vi "Load user settings.vi"(8 "error in (no error)":errorcluster, 11 "Test Framework in":refnum<class "Test Framework.lvclass">) -> (0 "error out":errorcluster, 2 "Canceled":bool, 3 "Test Framework out":refnum<class "Test Framework.lvclass">)   [LabVIEW 2020, in "Test Framework.lvclass"]
uses:
  Test Framework.lvclass
panel:
  in  "Cancel Button":bool
  in  "OK Button":bool caption="Restarts the framework"
  in  "User system setting file":path
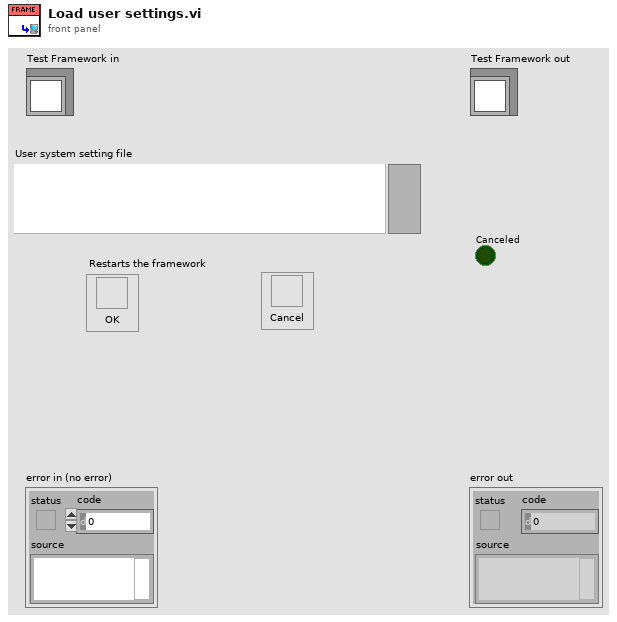
[diagram p1: front panel]
types:
  T1 = cluster{"Restart?":bool, "User system setting file":path}
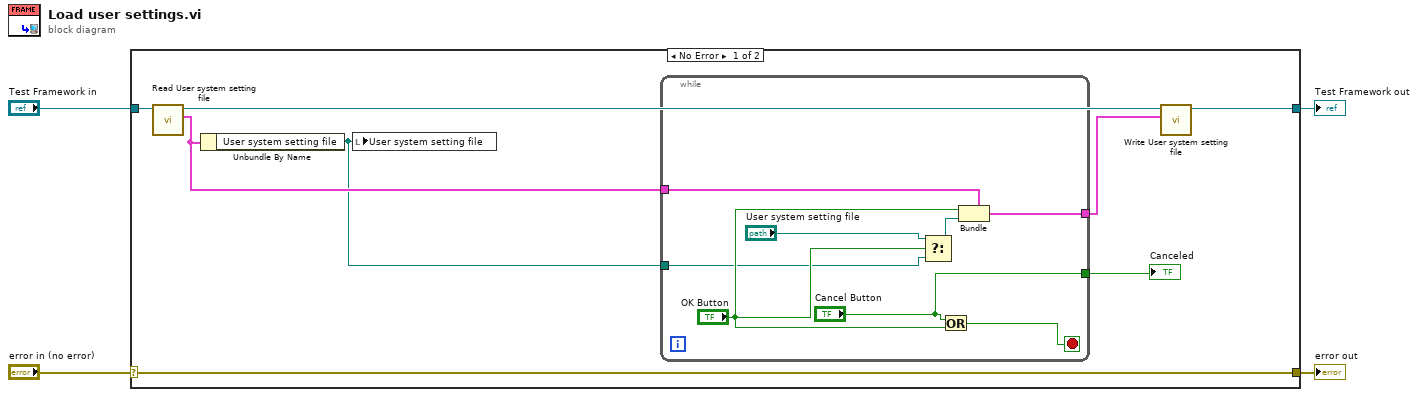
[diagram p0: block diagram]
diagram:
  n1 = case shown="No Error" "error in (no error)" {
    selector: "error in (no error)" -> [w12 w22]
    tunnel: [w12 w22] -> w3
    tunnel: [w9 w21] -> w1
    tunnel: "Test Framework in" -> [w11 w21]
    frame No Error {
      n2 = call-dynamic "Read User system setting file.vi"("Test Framework in"=w11) -> ("User system setting file"=w8:T1, "Test Framework out"=w10:refnum<class "Test Framework.lvclass">)  [unwired: 9 in]
      n3 = Unbundle By Name(w8) -> ("User system setting file"=w6:path)
      n4 = local write "User system setting file"(w6) -> ()
      n5 = while {
        tunnel: w8 -> [w20]
        tunnel: [w19] -> w7
        tunnel: w6 -> [w16]
        tunnel: ["Cancel Button"] -> w5
        stop <- w18 stop-if-true
        n6 = Select(t="User system setting file", s="OK Button", f=w16) -> (s? t:f=w14:path)
        n7 = Or(x="Cancel Button", y="OK Button") -> (x .or. y?=w18:bool)
        n8 = Bundle(cluster=w20, "Restart?"="OK Button", "User system setting file"=w14) -> (w19:T1)
      }
      "Canceled" <- w5
      n9 = call-dynamic "Write User system setting file.vi"("User system setting file"=w7, "Test Framework in"=w10) -> ("Test Framework out"=w9:refnum<class "Test Framework.lvclass">)  [unwired: 9 in]
    }
    frame Error {
    }
  }
  "error out" <- w3
  "Test Framework out" <- w1
